vi "tcp client module.vi"(8 "error in":errorcluster, 11 "name":string) -> (0 "error out":errorcluster)   [LabVIEW 2013]
doc: "# #############################################################################\n# ATTENTION\n# #############################################################################\n#\n# This software is for guidance only. It is provided \"as is\".\n# It only aims at providing coding information to the customer in order for\n# them to save time. As a result no warranties, whether express, implied or\n# statutory, including, but not limited to implied warranties of\n# merchantability and fitness for a particular purpose apply to this software.\n# A·P·E Angewandte Physik und Elektronik GmbH shall not be held liable for any\n# direct, indirect or consequential damages with respect to any claims arising\n# from the content of such sourcecode and/or the use made by customers of the\n# coding information contained herein in connection with their products.\n#\n# #############################################################################"
uses:
  queue control/queue cluster.ctl
  cluster/module cluster.ctl
panel:
  out "STOP":bool=TRUE
  in  "connect":bool
  in  "port":i32
  in  "ip":string
  out "read":string
  in  "query":bool
  in  "CMD":string="*idn?\n" caption="Command"
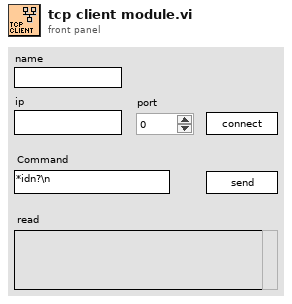
[diagram p1: front panel]
types:
  T1 = typedef "module cluster.ctl" = cluster{"connection ID":refnum<k5>, "ip":string, "port":u32, "termination":string, "write":string, "read":string, "connected":bool}
  T2 = typedef "queue cluster.ctl" = cluster{"command":string, "data":variant}
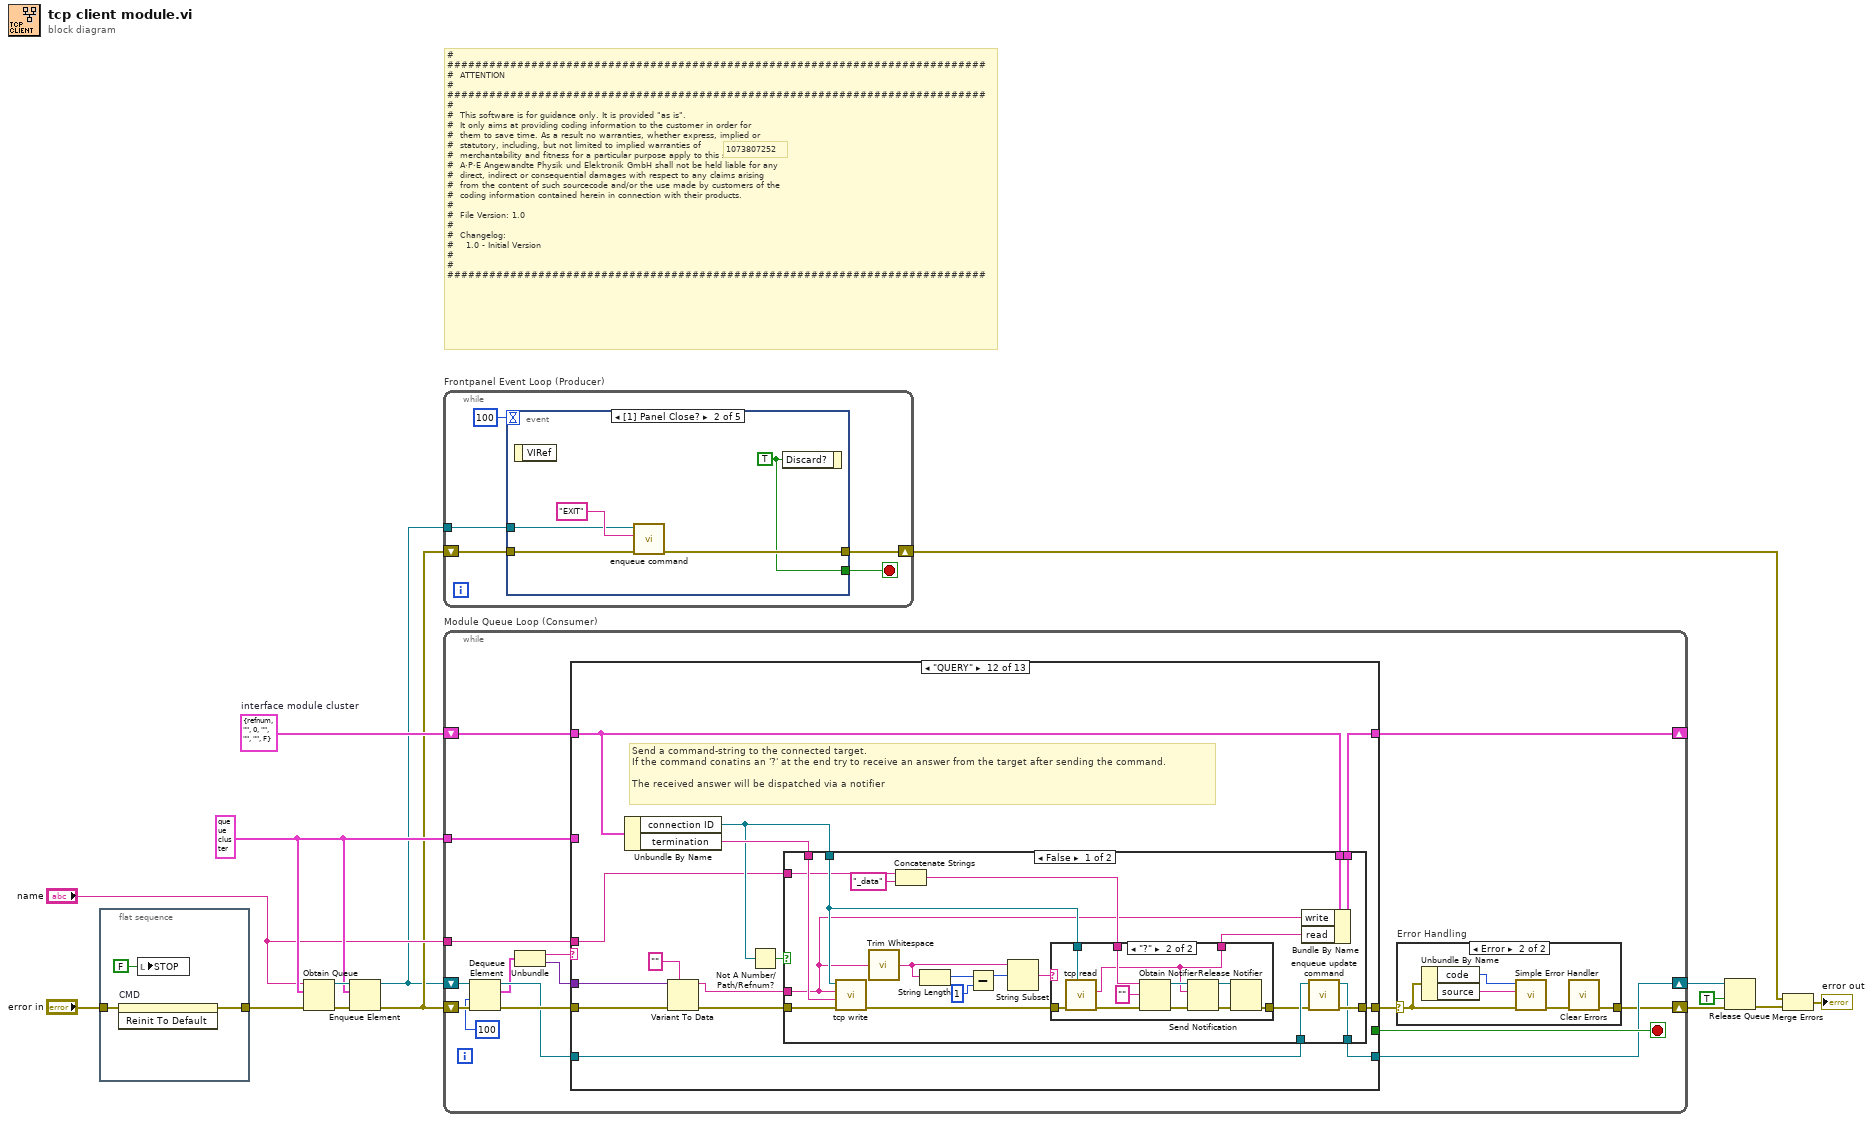
[diagram p0: block diagram]
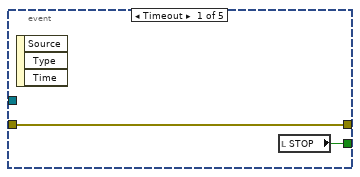
[diagram p2: hidden frame]
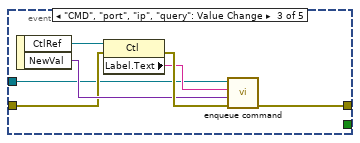
[diagram p3: hidden frame]
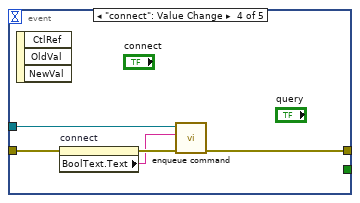
[diagram p4: hidden frame]
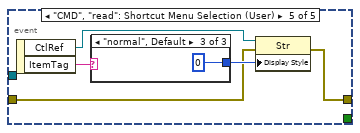
[diagram p5: hidden frame]
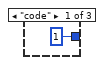
[diagram p6: hidden frame]
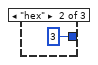
[diagram p7: hidden frame]
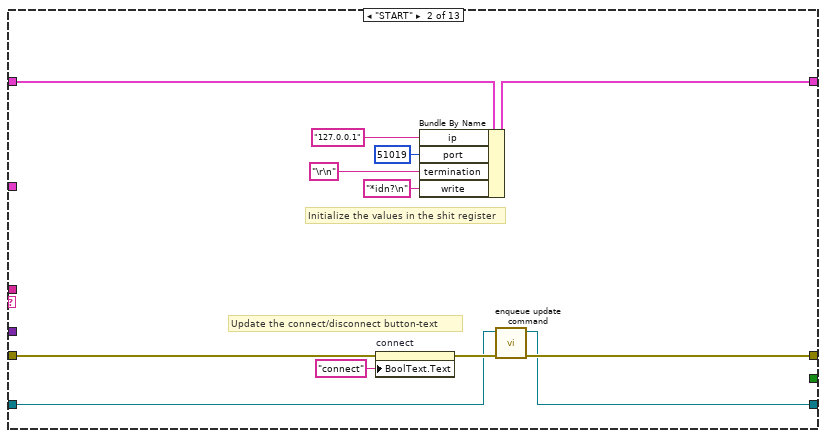
[diagram p10: hidden frame]
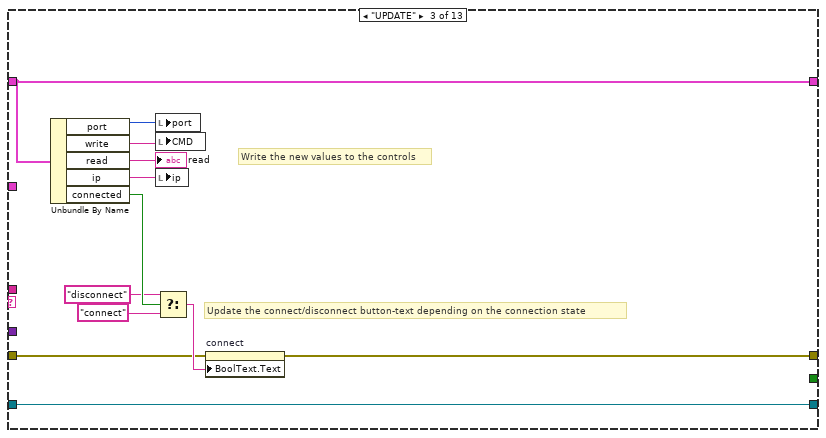
[diagram p11: hidden frame]
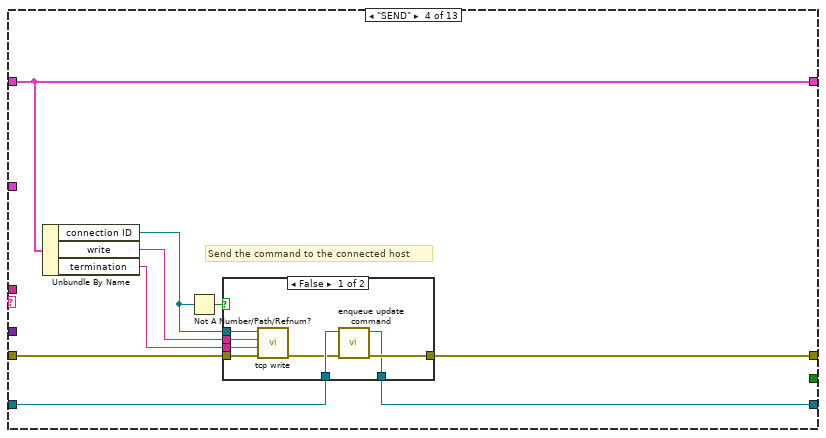
[diagram p12: hidden frame]
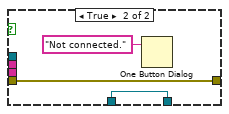
[diagram p13: hidden frame]
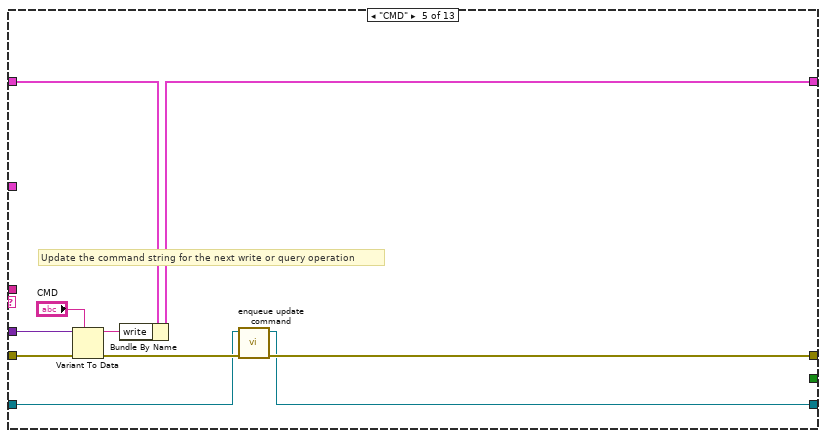
[diagram p14: hidden frame]
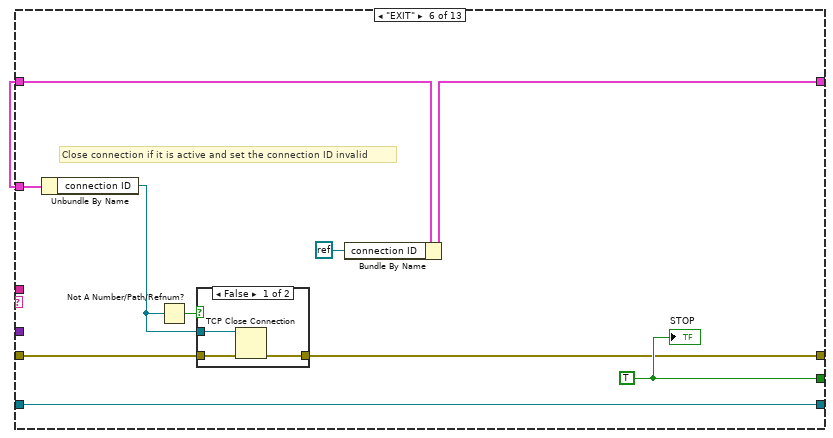
[diagram p15: hidden frame]
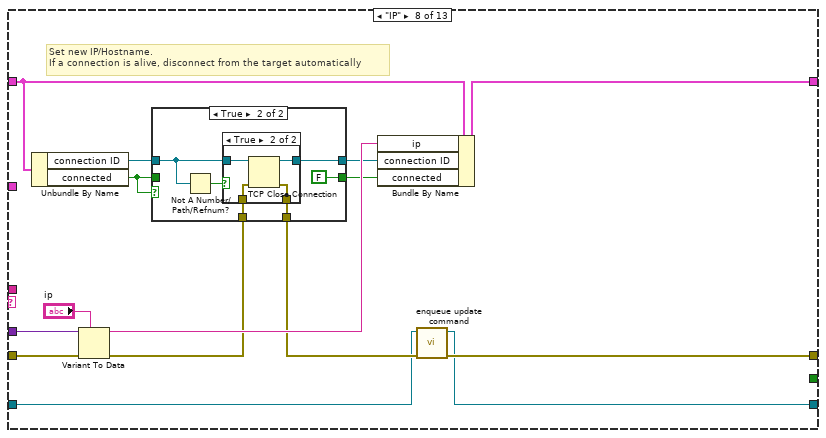
[diagram p18: hidden frame]
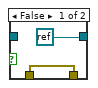
[diagram p20: hidden frame]
diagram:
  w7 = T1 {"connection ID"=refnum, "ip"="", "port"=0, "termination"="", "write"="", "read"="", "connected"=FALSE}  # interface module cluster
  w9 = T2 {"command"="START", "data"=variant} ("QDSM Element")
  # "# #############################################################################\n#  ATTENTION\n# #############################################################################\n#\n#  This software is for guidance only. It is provided \"as is\".\n#  It only aims at providing coding information to the customer in order for\n#  them to save time. As a result no warranties, whether express, implied or\n#  statutory, including, but not limited to implied warranties of\n#  merchantability and fitness for a particular purpose apply to this software.\n#  A·P·E Angewandte Physik und Elektronik GmbH shall not be held liable for any\n#  direct, indirect or consequential damages with respect to any claims arising\n#  from the content of such sourcecode and/or the use made by customers of the\n#  coding information contained herein in connection with their products.\n#\n#  File Version: 1.0\n#\n#  Changelog:\n#    1.0 - Initial Version\n#\n# #############################################################################"
  # "1073807252"
  n1 = flat-sequence {
    tunnel: "error in" -> [w16]
    tunnel: [w17] -> w1
    frame #0 {
      n2 = invoke on="CMD" class="Str" method="Reinit To Default"(error in=w16) -> (error out=w17:errorcluster)  [unwired: 2 in, 2 out]
      n3 = local write "STOP"(FALSE ("STOP")) -> ()
    }
  }
  n4 = Obtain Queue(name (unnamed)="name", element data type=w9, error in (no error)=w1) -> (queue out=w10:refnum<queue>, error out=w11:errorcluster)  [unwired: 2 in, 1 out]
  n5 = Enqueue Element(queue=w10, element=w9, error in (no error)=w11) -> (queue out=w5:refnum<queue>, error out=w6:errorcluster)  [unwired: 1 in, 1 out]
  n6 = while "Frontpanel Event Loop (Producer)" {
    tunnel: w5 -> [w22]
    shift-right: [w20] -> w3
    shift-left: w6 -> [w23]
    stop <- w19 stop-if-true
    n7 = event shown="[1] Panel Close?" {
      selector: _ -> [_ _ _ _ _]
      dyn-events: _ -> [_ _ _ _ _]
      timeout: 100 -> [_ _ _ _ _]
      tunnel: w23 -> [w25 w27 w32 w39 w43]
      tunnel: [w25 w30 w35 w41 w46] -> w20
      tunnel: w22 -> [_ w28 w31 w38 _]
      tunnel: [w24 w26 _ _ _] -> w19
      event Timeout {
        n8 = event-data() -> ()  [unwired: 4 out]
        n9 = local read "STOP"() -> (w24:bool)
      }
      event Panel Close? {
        w26 = TRUE ("Discard?")
        n10 = event-data() -> ()  [unwired: 2 out]
        n11 = call "enqueue command.vi"("error in"=w27, "Command"="EXIT" ("command"), "Queue in"=w28) -> ("error out"=w30:errorcluster)  [unwired: 7 in, 1 out]
        n12 = event-data("Discard?"=w26) -> ()  [unwired: 1 in, 1 out]
      }
      event "CMD", "port", "ip", "query": Value Change {
        n13 = event-data() -> ("CtlRef"=w37:refnum<vi>, "NewVal"=w33:variant)  [unwired: 1 out]
        n14 = property class="Ctl"(reference=w37, error in=w32) -> (error out=w36:errorcluster, "Label.Text"=w34:string)  [unwired: 1 out]
        n15 = call "enqueue command.vi"("error in"=w36, "Data"=w33, "Command"=w34, "Queue in"=w31) -> ("error out"=w35:errorcluster)  [unwired: 6 in, 1 out]
      }
      event "connect": Value Change {
        n16 = event-data() -> ()  [unwired: 4 out]
        n17 = property on="connect" class="Bool"(error in=w39) -> (error out=w42:errorcluster, "BoolText.Text"=w40:string)  [unwired: 1 in, 1 out]
        n18 = call "enqueue command.vi"("error in"=w42, "Command"=w40, "Queue in"=w38) -> ("error out"=w41:errorcluster)  [unwired: 7 in, 1 out]
      }
      event "CMD", "read": Shortcut Menu Selection (User) {
        n19 = event-data() -> ("CtlRef"=w44:refnum<vi>, "ItemTag"=w47:string)  [unwired: 1 out]
        n20 = case shown="\"normal\", Default" w47 {
          tunnel: [u32 1 ("Display Style") u32 3 ("Display Style") u32 0 ("Display Style")] -> w45
          frame "code" {
          }
          frame "hex" {
          }
          frame "normal", Default {
          }
        }
        n21 = property class="Str"(reference=w44, error in=w43, "Display Style"=w45) -> (error out=w46:errorcluster)  [unwired: 1 out]
      }
    }
  }
  n22 = while "Module Queue Loop (Consumer)" {
    shift-right: [w53] -> w13
    shift-left: w6 -> [w61]
    shift-right: [w60] -> _
    shift-left: w7 -> [w63]
    tunnel: w9 -> [w62]
    tunnel: "name" -> [w59]
    shift-right: [w55] -> w14
    shift-left: w5 -> [w58]
    stop <- w66 stop-if-true
    n23 = Dequeue Element(queue=w58, timeout in ms (-1)=100 ("timeout out"), error in (no error)=w61) -> (queue out=w64:refnum<queue>, element=w57:T2, error out=w65:errorcluster)  [unwired: 1 out]
    n24 = Unbundle(w57) -> ("command"=w51:string, "data"=w56:variant)
    n25 = case shown="\"QUERY\"" w51 {
      tunnel: w64 -> [w74 w79 w89 w102 w121 w137 w143 w147 w177 w210 w232 w257 w300]
      tunnel: [_ _ _ _ _ w138 _ _ _ _ _ _ _] -> w66
      tunnel: w65 -> [w73 w77 w90 w107 w125 w131 w144 w157 w189 w222 w235 w251 w307]
      tunnel: [w73 w80 w88 w104 w122 w130 w144 w149 w179 w206 w233 w258 w301] -> w52
      tunnel: w63 -> [w75 w87 w97 w108 w129 w136 w145 w156 w184 w223 w239 w261 w308]
      tunnel: w62 -> [_ _ _ _ _ _ _ _ _ _ _ _ _]
      tunnel: [w75 w85 w97 w108 w128 w135 w145 w159 w185 w221 w238 w260 w306] -> w60
      tunnel: [w74 w78 w89 w103 w120 w137 w143 w146 w176 w207 w231 w256 w299] -> w55
      tunnel: w59 -> [_ _ _ _ _ _ _ _ _ _ _ w253 _]
      tunnel: w56 -> [_ _ _ _ w124 _ _ w151 w182 _ _ w250 w305]
      frame "", Default {
        # "No action requested / Idle-State / Unknown command received"
      }
      frame "START" {
        # "Update the connect/disconnect button-text"
        # "Initialize the values in the shit register"
        n26 = property on="connect" class="Bool"(error in=w77, "BoolText.Text"="connect" ("Boolean Text.Text")) -> (error out=w81:errorcluster)  [unwired: 1 in, 1 out]
        n27 = Bundle By Name(cluster=w87, "ip"="127.0.0.1", "port"=u32 51019, "termination"="\r\n", "write"="*idn?\n") -> (w85:T1)
        n28 = call "enqueue update command.vi"("error in"=w81, "Queue in"=w79) -> ("error out"=w80:errorcluster, "Queue out"=w78:refnum<queue>)  [unwired: 8 in]
      }
      frame "UPDATE" {
        # "Update the connect/disconnect button-text depending on the connection state"
        # "Write the new values to the controls"
        n29 = Unbundle By Name(w97) -> ("port"=w95:u32, "write"=w98:string, "read"=→"read":string, "ip"=w96:string, "connected"=w94:bool)
        n30 = local write "port"(w95) -> ()
        n31 = local write "CMD"(w98) -> ()
        n32 = local write "ip"(w96) -> ()
        n33 = Select(t="disconnect", s=w94, f="connect" ("Boolean Text.Text")) -> (s? t:f=w91:string)
        n34 = property on="connect" class="Bool"(error in=w90, "BoolText.Text"=w91) -> (error out=w88:errorcluster)  [unwired: 1 in, 1 out]
      }
      frame "SEND" {
        # "Send the command to the connected host"
        n35 = Unbundle By Name(w108) -> ("connection ID"=w101:refnum<k5>, "write"=w105:string, "termination"=w106:string)
        n36 = Not A Number/Path/Refnum?(number/path/refnum=w101) -> (NaN/Path/Refnum?=w100:bool)
        n37 = case shown="False" w100 {
          tunnel: w107 -> [w116 w118]
          tunnel: w106 -> [w115 _]
          tunnel: w105 -> [w114 _]
          tunnel: [w113 w118] -> w104
          tunnel: [w112 w119] -> w103
          tunnel: w102 -> [w111 w119]
          tunnel: w101 -> [w109 _]
          frame False {
            n38 = call "tcp write.vi"("error in"=w116, "termination"=w115, "Data"=w114, "Connection in"=w109) -> ("error out"=w110:errorcluster)  [unwired: 7 in]
            n39 = call "enqueue update command.vi"("error in"=w110, "Queue in"=w111) -> ("error out"=w113:errorcluster, "Queue out"=w112:refnum<queue>)  [unwired: 8 in]
          }
          frame True {
            n40 = One Button Dialog(message="Not connected.") -> ()  [unwired: 1 in, 1 out]
          }
        }
      }
      frame "CMD" {
        # "Update the command string for the next write or query operation"
        n41 = Variant To Data(error in=w125, type="CMD", Variant=w124) -> (data=w126:string, error out=w123:errorcluster)
        n42 = Bundle By Name(cluster=w129, "write"=w126) -> (w128:T1)
        n43 = call "enqueue update command.vi"("error in"=w123, "Queue in"=w121) -> ("error out"=w122:errorcluster, "Queue out"=w120:refnum<queue>)  [unwired: 8 in]
      }
      frame "EXIT" {
        w138 = TRUE
        # "Close connection if it is active and set the connection ID invalid"
        n44 = Unbundle By Name(w136) -> ("connection ID"=w132:refnum<k5>)
        n45 = Not A Number/Path/Refnum?(number/path/refnum=w132) -> (NaN/Path/Refnum?=w133:bool)
        n46 = case shown="False" w133 {
          tunnel: w131 -> [w141 w142]
          tunnel: [w140 w142] -> w130
          tunnel: w132 -> [w139 _]
          frame False {
            n47 = TCP Close Connection(connection ID=w139, error in (no error)=w141) -> (error out=w140:errorcluster)  [unwired: 1 in, 1 out]
          }
          frame True {
          }
        }
        n48 = Bundle By Name(cluster=w136, "connection ID"=refnum<k0> refnum) -> (w135:T1)
        "STOP" <- w138
      }
      frame "--------- USER COMMANDS BELOW ---------" {
      }
      frame "IP" {
        # "Set new IP/Hostname.\nIf a connection is alive, disconnect from the target automatically"
        n49 = Unbundle By Name(w156) -> ("connection ID"=w155:refnum<k5>, "connected"=w152:bool)
        n50 = Variant To Data(error in=w157, type="ip", Variant=w151) -> (data=w158:string, error out=w150:errorcluster)
        n51 = case shown="True" w152 {
          tunnel: w155 -> [w162 w169]
          tunnel: [w162 w167] -> w154
          tunnel: [w163 FALSE] -> w153
          tunnel: w152 -> [w163 _]
          tunnel: w150 -> [w161 w165]
          tunnel: [w161 w164] -> w148
          frame False {
          }
          frame True {
            n52 = Not A Number/Path/Refnum?(number/path/refnum=w169) -> (NaN/Path/Refnum?=w168:bool)
            n53 = case shown="True" w168 {
              tunnel: w169 -> [_ w175]
              tunnel: [refnum<k0> refnum w174] -> w167
              tunnel: w165 -> [w170 w173]
              tunnel: [w170 w172] -> w164
              frame False {
              }
              frame True {
                n54 = TCP Close Connection(connection ID=w175, error in (no error)=w173) -> (connection ID out=w174:refnum<k5>, error out=w172:errorcluster)  [unwired: 1 in]
              }
            }
          }
        }
        n55 = Bundle By Name(cluster=w156, "ip"=w158, "connection ID"=w154, "connected"=w153) -> (w159:T1)
        n56 = call "enqueue update command.vi"("error in"=w148, "Queue in"=w147) -> ("error out"=w149:errorcluster, "Queue out"=w146:refnum<queue>)  [unwired: 8 in]
      }
      frame "PORT" {
        # "Set new TCP Port.\nIf a connection is alive, disconnect from the target automatically"
        n57 = Unbundle By Name(w184) -> ("connection ID"=w188:refnum<k5>, "connected"=w181:bool)
        n58 = Variant To Data(error in=w189, type="port", Variant=w182) -> (data=w183:i32, error out=w180:errorcluster)
        n59 = case shown="True" w181 {
          selector: w181 -> [w192 _]
          tunnel: w188 -> [w193 w199]
          tunnel: [w193 w197] -> w187
          tunnel: [w192 FALSE] -> w186
          tunnel: w180 -> [w191 w195]
          tunnel: [w191 w194] -> w178
          frame False {
          }
          frame True {
            n60 = Not A Number/Path/Refnum?(number/path/refnum=w199) -> (NaN/Path/Refnum?=w198:bool)
            n61 = case shown="True" w198 {
              tunnel: w199 -> [_ w205]
              tunnel: [refnum<k0> refnum w204] -> w197
              tunnel: w195 -> [w200 w203]
              tunnel: [w200 w202] -> w194
              frame False {
              }
              frame True {
                n62 = TCP Close Connection(connection ID=w205, error in (no error)=w203) -> (connection ID out=w204:refnum<k5>, error out=w202:errorcluster)  [unwired: 1 in]
              }
            }
          }
        }
        n63 = Bundle By Name(cluster=w184, "port"=w183, "connection ID"=w187, "connected"=w186) -> (w185:T1)
        n64 = call "enqueue update command.vi"("error in"=w178, "Queue in"=w177) -> ("error out"=w179:errorcluster, "Queue out"=w176:refnum<queue>)  [unwired: 8 in]
      }
      frame "CONNECT" {
        # "Try to establish a TCP Connection to the specified target\nIf a connection is still alive, close this one first"
        n65 = Unbundle By Name(w223) -> ("ip"=w219:string, "port"=w218:u32, "connection ID"=w220:refnum<k5>)
        n66 = Not A Number/Path/Refnum?(number/path/refnum=w220) -> (NaN/Path/Refnum?=w215:bool)
        n67 = case shown="False" w215 {
          tunnel: w222 -> [w229 w230]
          tunnel: [w228 w230] -> w214
          tunnel: w220 -> [w227 _]
          frame False {
            n68 = TCP Close Connection(connection ID=w227, error in (no error)=w229) -> (error out=w228:errorcluster)  [unwired: 1 in, 1 out]
          }
          frame True {
          }
        }
        n69 = TCP Open Connection(address=w219, remote port or service name=w218, timeout ms (60000)=500, error in (no error)=w214) -> (connection ID=w217:refnum<k5>, error out=w209:errorcluster)  [unwired: 1 in]
        n70 = Unbundle By Name(w209) -> ("code"=w208:i32)
        n71 = Not A Number/Path/Refnum?(number/path/refnum=w217) -> (NaN/Path/Refnum?=w212:bool)
        n72 = Not(x=w212) -> (.not. x?=w216:bool)
        n73 = case shown="56, 63" w208 {
          tunnel: [w224 w225] -> w211
          tunnel: w209 -> [w224 w226]
          frame Default {
          }
          frame 56, 63 {
            n74 = call <vilib>:"Clear Errors.vi"("error in (no error)"=w226) -> ("error out"=w225:errorcluster)  [unwired: 5 in, 1 out]
          }
        }
        n75 = Bundle By Name(cluster=w223, "connection ID"=w217, "connected"=w216) -> (w221:T1)
        n76 = call "enqueue update command.vi"("error in"=w211, "Queue in"=w210) -> ("error out"=w206:errorcluster, "Queue out"=w207:refnum<queue>)  [unwired: 8 in]
      }
      frame "DISCONNECT" {
        # "Terminate the currently active connection"
        n77 = Unbundle By Name(w239) -> ("connection ID"=w240:refnum<k5>)
        n78 = Not A Number/Path/Refnum?(number/path/refnum=w240) -> (NaN/Path/Refnum?=w241:bool)
        n79 = case shown="False" w241 {
          tunnel: w235 -> [w245 w247]
          tunnel: [w244 w247] -> w234
          tunnel: w240 -> [w243 w246]
          tunnel: [w242 w246] -> w237
          frame False {
            n80 = TCP Close Connection(connection ID=w243, error in (no error)=w245) -> (connection ID out=w242:refnum<k5>, error out=w244:errorcluster)  [unwired: 1 in]
          }
          frame True {
          }
        }
        n81 = Bundle By Name(cluster=w239, "connection ID"=w237, "connected"=FALSE) -> (w238:T1)
        n82 = call "enqueue update command.vi"("error in"=w234, "Queue in"=w232) -> ("error out"=w233:errorcluster, "Queue out"=w231:refnum<queue>)  [unwired: 8 in]
      }
      frame "QUERY" {
        # "Send a command-string to the connected target. \nIf the command conatins an '?' at the end try to receive an answer from the target after sending the command.\n\nThe received answer will be dispatched via a notifier"
        n83 = Unbundle By Name(w261) -> ("connection ID"=w255:refnum<k5>, "termination"=w259:string)
        n84 = Variant To Data(error in=w251, type="", Variant=w250) -> (data=w249:string, error out=w252:errorcluster)
        n85 = Not A Number/Path/Refnum?(number/path/refnum=w255) -> (NaN/Path/Refnum?=w254:bool)
        n86 = case shown="False" w254 {
          tunnel: w261 -> [w281 w294]
          tunnel: [w280 w294] -> w260
          tunnel: w252 -> [w278 w295]
          tunnel: w255 -> [w273 _]
          tunnel: w259 -> [w274 _]
          tunnel: [w277 w295] -> w258
          tunnel: w257 -> [w276 w296]
          tunnel: [w275 w296] -> w256
          tunnel: w253 -> [w272 _]
          tunnel: w249 -> [w262 _]
          frame False {
            n87 = call "tcp write.vi"("error in"=w278, "termination"=w274, "Data"=w262, "Connection in"=w273) -> ("error out"=w279:errorcluster)  [unwired: 7 in]
            n88 = call <vilib>:"Trim Whitespace.vi"("string"=w262) -> ("trimmed string"=w264:string)  [unwired: 1 in]
            n89 = Concatenate Strings(w272, "_data" ("string")) -> (w271:string)
            n90 = String Length(string=w264) -> (length=w266:i32)
            n91 = Subtract(x=w266, y=1) -> (x-y=w265:i32)
            n92 = String Subset(string=w264, offset (0)=w265) -> (substring=w263:string)  [unwired: 1 in]
            n93 = case shown="\"?\"" w263 {
              tunnel: w279 -> [w282 w293]
              tunnel: w273 -> [_ w292]
              tunnel: w271 -> [_ w289]
              tunnel: [_ w286] -> w269
              tunnel: [w282 w283] -> w268
              frame Default {
              }
              frame "?" {
                n94 = call "tcp read.vi"("Connection in"=w292, "error in"=w293) -> ("error out"=w291:errorcluster, "Data"=w286:string)  [unwired: 8 in]
                n95 = Obtain Notifier(name (unnamed)=w289, notification data type="", error in (no error)=w291) -> (notifier out=w288:refnum<notifier>, error out=w287:errorcluster)  [unwired: 1 in, 1 out]
                n96 = Send Notification(notification=w286, notifier=w288, error in (no error)=w287) -> (notifier out=w285:refnum<notifier>, error out=w284:errorcluster)
                n97 = Release Notifier(notifier=w285, error in (no error)=w284) -> (error out=w283:errorcluster)  [unwired: 1 in, 2 out]
              }
            }
            n98 = Bundle By Name(cluster=w281, "write"=w262, "read"=w269) -> (w280:T1)
            n99 = call "enqueue update command.vi"("error in"=w268, "Queue in"=w276) -> ("error out"=w277:errorcluster, "Queue out"=w275:refnum<queue>)  [unwired: 8 in]
          }
          frame True {
            # "Not connected."
          }
        }
      }
      frame "WRITE" {
        w302 = "" ("termination")
        # "Write a command to the target, but don't try to receive an answer"
        n100 = Unbundle By Name(w308) -> ("connection ID"=w297:refnum<k5>)
        n101 = Variant To Data(error in=w307, type=w302, Variant=w305) -> (data=w303:string, error out=w304:errorcluster)
        n102 = Not A Number/Path/Refnum?(number/path/refnum=w297) -> (NaN/Path/Refnum?=w298:bool)
        n103 = case shown="False" w298 {
          tunnel: w308 -> [w319 w320]
          tunnel: [w318 w320] -> w306
          tunnel: w304 -> [w316 w323]
          tunnel: w297 -> [w315 _]
          tunnel: w303 -> [w314 _]
          tunnel: w302 -> [w313 _]
          tunnel: [w311 w323] -> w301
          tunnel: w300 -> [w310 w322]
          tunnel: [w309 w322] -> w299
          frame False {
            n104 = call "tcp write.vi"("error in"=w316, "termination"=w313, "Data"=w314, "Connection in"=w315) -> ("error out"=w312:errorcluster)  [unwired: 7 in]
            n105 = Bundle By Name(cluster=w319, "write"=w314, "read"="") -> (w318:T1)
            n106 = call "enqueue update command.vi"("error in"=w312, "Queue in"=w310) -> ("error out"=w311:errorcluster, "Queue out"=w309:refnum<queue>)  [unwired: 8 in]
          }
          frame True {
            n107 = One Button Dialog(message="Not connected.") -> ()  [unwired: 1 in, 1 out]
          }
        }
      }
    }
    n108 = case "Error Handling" shown="Error" w52 {
      selector: w52 -> [w67 w71]
      tunnel: [w67 w68] -> w53
      frame No Error {
      }
      frame Error {
        n109 = Unbundle By Name(w71) -> ("code"=w70:i32, "source"=w69:string)
        n110 = call <vilib>:"Simple Error Handler.vi"("error code (no error:0)"=w70, "error source (\" \")"=w69, "error in (no error)"=w71) -> ("error out"=w72:errorcluster)  [unwired: 2 in, 4 out]
        n111 = call <vilib>:"Clear Errors.vi"("error in (no error)"=w72) -> ("error out"=w68:errorcluster)  [unwired: 5 in, 1 out]
      }
    }
  }
  n112 = Release Queue(queue=w14, force destroy? (F)=TRUE, error in (no error)=w13) -> (error out=w12:errorcluster)  [unwired: 2 out]
  n113 = Merge Errors(w3, w12) -> (→"error out":errorcluster)
